vi "Yellow to Red 2.vi"   [LabVIEW 2019]
uses:
  Global Var.vi
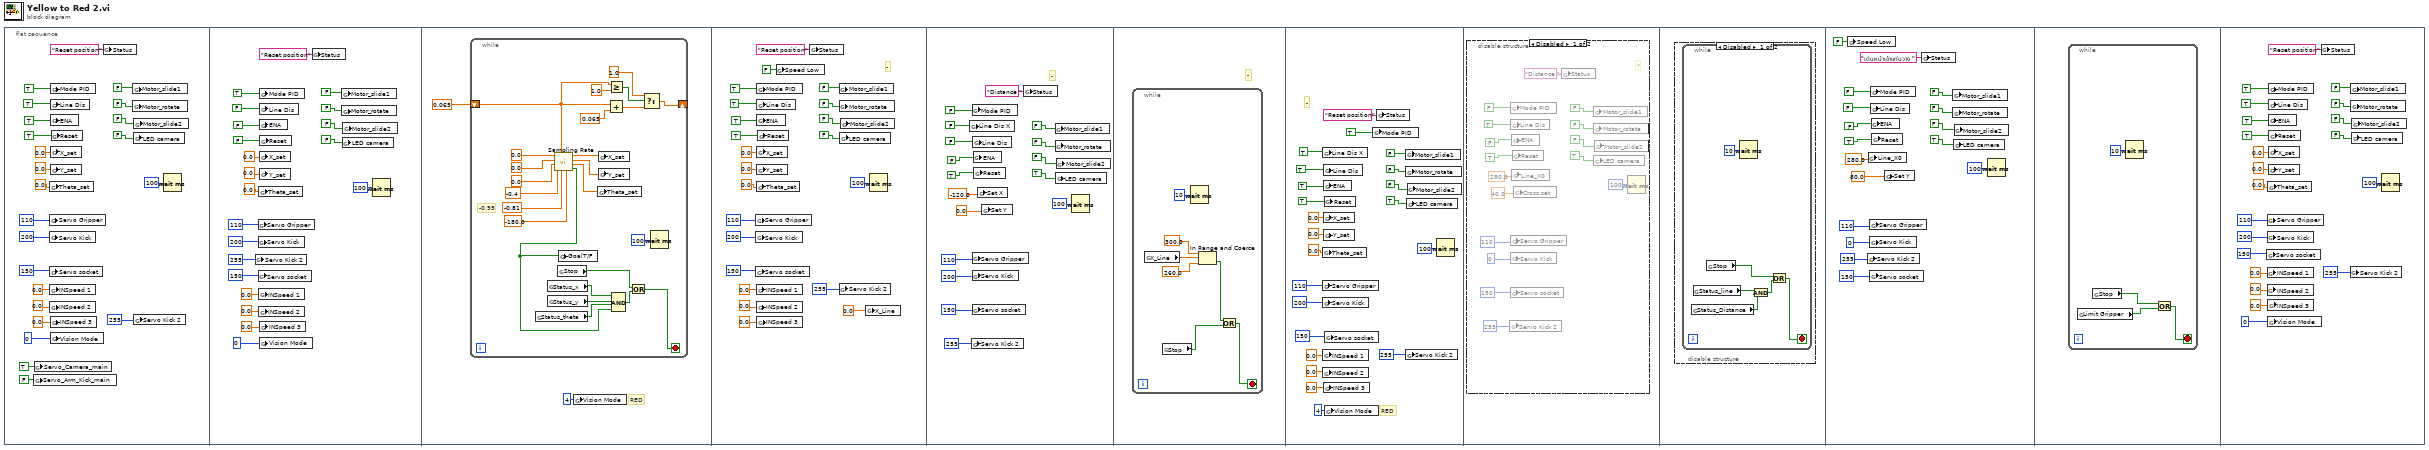
[diagram p0: block diagram]
diagram:
  n1 = flat-sequence {
    frame #0 {
      n2 = global write "Global Var.vi" "Servo_Arm_Kick_main"(FALSE ("Mode PID")) -> ()
      n3 = global write "Global Var.vi" "Servo_Camera_main"(TRUE ("Mode PID")) -> ()
      n4 = global write "Global Var.vi" "Servo Gripper"(u8 110 ("Servo Camera")) -> ()
      n5 = global write "Global Var.vi" "Servo Kick"(u8 200 ("Servo Camera")) -> ()
      n6 = global write "Global Var.vi" "Servo socket"(u8 150 ("Servo Camera")) -> ()
      n7 = global write "Global Var.vi" "Theta_set"(0.0 ("Theta_set")) -> ()
      n8 = global write "Global Var.vi" "INSpeed 1"(0.0 ("X_set")) -> ()
      n9 = global write "Global Var.vi" "INSpeed 2"(0.0 ("Y_set")) -> ()
      n10 = global write "Global Var.vi" "Mode PID"(TRUE ("Mode PID")) -> ()
      n11 = global write "Global Var.vi" "Line Dis"(TRUE ("Mode PID")) -> ()
      n12 = global write "Global Var.vi" "ENA"(TRUE ("ENA")) -> ()
      n13 = global write "Global Var.vi" "X_set"(0.0 ("X_set")) -> ()
      n14 = global write "Global Var.vi" "Y_set"(0.0 ("Y_set")) -> ()
      n15 = global write "Global Var.vi" "INSpeed 3"(0.0 ("Theta_set")) -> ()
      n16 = global write "Global Var.vi" "Vision Mode"(i16 0 ("Vision Mode")) -> ()
      n17 = global write "Global Var.vi" "Reset"(TRUE ("ENA")) -> ()
      n18 = global write "Global Var.vi" "Status"("Reset position" ("Status")) -> ()
      n19 = global write "Global Var.vi" "Motor_slide1"(FALSE ("Mode PID")) -> ()
      n20 = global write "Global Var.vi" "Motor_rotate"(FALSE ("ENA")) -> ()
      n21 = global write "Global Var.vi" "LED camera"(FALSE ("LED camera")) -> ()
      n22 = global write "Global Var.vi" "Motor_slide2"(FALSE ("ENA")) -> ()
      n23 = global write "Global Var.vi" "Servo Kick 2"(u8 255 ("Servo Camera")) -> ()
      n24 = Wait (ms)(milliseconds to wait=u32 100) -> ()  [unwired: 1 out]
    }
    frame #1 {
      n25 = global write "Global Var.vi" "Servo Kick 2"(u8 255 ("Servo Camera")) -> ()
      n26 = global write "Global Var.vi" "Servo Gripper"(u8 110 ("Servo Camera")) -> ()
      n27 = global write "Global Var.vi" "Servo Kick"(u8 200 ("Servo Camera")) -> ()
      n28 = global write "Global Var.vi" "Servo socket"(u8 150 ("Servo Camera")) -> ()
      n29 = global write "Global Var.vi" "Theta_set"(0.0 ("Theta_set")) -> ()
      n30 = global write "Global Var.vi" "INSpeed 1"(0.0 ("X_set")) -> ()
      n31 = global write "Global Var.vi" "INSpeed 2"(0.0 ("Y_set")) -> ()
      n32 = global write "Global Var.vi" "Mode PID"(TRUE ("Mode PID")) -> ()
      n33 = global write "Global Var.vi" "Line Dis"(FALSE ("Mode PID")) -> ()
      n34 = global write "Global Var.vi" "ENA"(FALSE ("ENA")) -> ()
      n35 = global write "Global Var.vi" "X_set"(0.0 ("X_set")) -> ()
      n36 = global write "Global Var.vi" "Y_set"(0.0 ("Y_set")) -> ()
      n37 = global write "Global Var.vi" "INSpeed 3"(0.0 ("Theta_set")) -> ()
      n38 = global write "Global Var.vi" "Vision Mode"(i16 0 ("Vision Mode")) -> ()
      n39 = global write "Global Var.vi" "Reset"(FALSE ("ENA")) -> ()
      n40 = global write "Global Var.vi" "Status"("Reset position" ("Status")) -> ()
      n41 = global write "Global Var.vi" "Motor_slide1"(FALSE ("Mode PID")) -> ()
      n42 = global write "Global Var.vi" "Motor_rotate"(FALSE ("ENA")) -> ()
      n43 = global write "Global Var.vi" "LED camera"(FALSE ("LED camera")) -> ()
      n44 = global write "Global Var.vi" "Motor_slide2"(FALSE ("ENA")) -> ()
      n45 = Wait (ms)(milliseconds to wait=u32 100) -> ()  [unwired: 1 out]
    }
    frame #2 {
      # "RED"
      n46 = while {
        shift-right: [w49] -> _
        shift-left: 0.065 -> [w47]
        stop <- w66 stop-if-true
        # "-0.95"
        n47 = global read "Global Var.vi" "Status_theta"() -> (w68:bool)
        n48 = global read "Global Var.vi" "Status_x"() -> (w69:bool)
        n49 = global read "Global Var.vi" "Status_y"() -> (w70:bool)
        n50 = call "Sampling Rate.vi"("input a1"=-180.0, "input y1"=-0.81, "T(0-1)"=w47, "input x1"=-0.4, "input a0"=0.0, "input y0"=0.0, "input x0"=0.0) -> ("GoalT/F"=w54:bool, "a_output"=w61:dbl, "y_output"=w62:dbl, "x_output"=w63:dbl)  [unwired: 1 in]
        n51 = global read "Global Var.vi" "Stop"() -> (w64:bool)
        n52 = global write "Global Var.vi" "GoalT/F"(w54) -> ()
        n53 = global write "Global Var.vi" "Theta_set"(w61) -> ()
        n54 = global write "Global Var.vi" "X_set"(w63) -> ()
        n55 = global write "Global Var.vi" "Y_set"(w62) -> ()
        n56 = Add(x=w47, y=0.065) -> (x+y=w52:dbl)
        n57 = Greater Or Equal?(x=w47, y=1.0) -> (x >= y?=w51:bool)
        n58 = Compound Arithmetic op=AND(w69, w70, w68, w54) -> (w65:bool)
        n59 = Or(x=w64, y=w65) -> (x .or. y?=w66:bool)
        n60 = Select(t=1.0, s=w51, f=w52) -> (s? t:f=w49:dbl)
        n61 = Wait (ms)(milliseconds to wait=u32 100) -> ()  [unwired: 1 out]
      }
      n62 = global write "Global Var.vi" "Vision Mode"(i16 4 ("Vision Mode")) -> ()
    }
    frame #3 {
      # "-"
      n63 = global write "Global Var.vi" "Servo Gripper"(u8 110 ("Servo Camera")) -> ()
      n64 = global write "Global Var.vi" "Servo Kick"(u8 200 ("Servo Camera")) -> ()
      n65 = global write "Global Var.vi" "Servo socket"(u8 150 ("Servo Camera")) -> ()
      n66 = global write "Global Var.vi" "Theta_set"(0.0 ("Theta_set")) -> ()
      n67 = global write "Global Var.vi" "INSpeed 1"(0.0 ("X_set")) -> ()
      n68 = global write "Global Var.vi" "INSpeed 2"(0.0 ("Y_set")) -> ()
      n69 = global write "Global Var.vi" "Mode PID"(TRUE ("Mode PID")) -> ()
      n70 = global write "Global Var.vi" "Line Dis"(TRUE ("Mode PID")) -> ()
      n71 = global write "Global Var.vi" "ENA"(TRUE ("ENA")) -> ()
      n72 = global write "Global Var.vi" "X_set"(0.0 ("X_set")) -> ()
      n73 = global write "Global Var.vi" "Y_set"(0.0 ("Y_set")) -> ()
      n74 = global write "Global Var.vi" "INSpeed 3"(0.0 ("Theta_set")) -> ()
      n75 = global write "Global Var.vi" "Reset"(TRUE ("ENA")) -> ()
      n76 = global write "Global Var.vi" "Speed Low"(FALSE ("Speed Low")) -> ()
      n77 = global write "Global Var.vi" "Status"("Reset position" ("Status")) -> ()
      n78 = global write "Global Var.vi" "Motor_slide1"(FALSE ("Mode PID")) -> ()
      n79 = global write "Global Var.vi" "Motor_rotate"(FALSE ("ENA")) -> ()
      n80 = global write "Global Var.vi" "Servo Kick 2"(u8 255 ("Servo Camera")) -> ()
      n81 = global write "Global Var.vi" "LED camera"(FALSE ("LED camera")) -> ()
      n82 = global write "Global Var.vi" "Motor_slide2"(FALSE ("ENA")) -> ()
      n83 = global write "Global Var.vi" "X_Line"(0.0 ("X_set")) -> ()
      n84 = Wait (ms)(milliseconds to wait=u32 100) -> ()  [unwired: 1 out]
    }
    frame #4 {
      # "-"
      n85 = global write "Global Var.vi" "Line Dis X"(FALSE ("Mode PID")) -> ()
      n86 = global write "Global Var.vi" "Servo Kick 2"(u8 255 ("Servo Camera")) -> ()
      n87 = global write "Global Var.vi" "Mode PID"(FALSE ("Mode PID")) -> ()
      n88 = global write "Global Var.vi" "Servo Gripper"(u8 110 ("Servo Camera")) -> ()
      n89 = global write "Global Var.vi" "Servo Kick"(u8 200 ("Servo Camera")) -> ()
      n90 = global write "Global Var.vi" "Servo socket"(u8 150 ("Servo Camera")) -> ()
      n91 = global write "Global Var.vi" "Line Dis"(FALSE ("Mode PID")) -> ()
      n92 = global write "Global Var.vi" "ENA"(FALSE ("ENA")) -> ()
      n93 = global write "Global Var.vi" "Reset"(TRUE ("ENA")) -> ()
      n94 = global write "Global Var.vi" "Set X"(-120.0 ("Y_set")) -> ()
      n95 = global write "Global Var.vi" "Set Y"(0.0 ("Y_set")) -> ()
      n96 = global write "Global Var.vi" "Status"("Distance " ("Status")) -> ()
      n97 = global write "Global Var.vi" "Motor_slide1"(FALSE ("Mode PID")) -> ()
      n98 = global write "Global Var.vi" "Motor_rotate"(FALSE ("ENA")) -> ()
      n99 = global write "Global Var.vi" "LED camera"(TRUE ("LED camera")) -> ()
      n100 = global write "Global Var.vi" "Motor_slide2"(FALSE ("ENA")) -> ()
      n101 = Wait (ms)(milliseconds to wait=u32 100) -> ()  [unwired: 1 out]
    }
    frame #5 {
      # "-"
      n102 = while {
        stop <- w115 stop-if-true
        n103 = global read "Global Var.vi" "X_Line"() -> (w113:dbl)
        n104 = global read "Global Var.vi" "Stop"() -> (w114:bool)
        n105 = Wait (ms)(milliseconds to wait=u32 10) -> ()  [unwired: 1 out]
        n106 = In Range and Coerce(upper limit=300.0, x=w113, lower limit=260.0) -> (In Range?=w110:bool)  [unwired: 1 out]
        n107 = Or(x=w110, y=w114) -> (x .or. y?=w115:bool)
      }
    }
    frame #6 {
      # "RED"
      # "-"
      n108 = global write "Global Var.vi" "Servo Gripper"(u8 110 ("Servo Camera")) -> ()
      n109 = global write "Global Var.vi" "Servo Kick"(u8 200 ("Servo Camera")) -> ()
      n110 = global write "Global Var.vi" "Line Dis X"(TRUE ("Mode PID")) -> ()
      n111 = global write "Global Var.vi" "Theta_set"(0.0 ("Theta_set")) -> ()
      n112 = global write "Global Var.vi" "INSpeed 1"(0.0 ("X_set")) -> ()
      n113 = global write "Global Var.vi" "INSpeed 2"(0.0 ("Y_set")) -> ()
      n114 = global write "Global Var.vi" "Line Dis"(TRUE ("Mode PID")) -> ()
      n115 = global write "Global Var.vi" "ENA"(TRUE ("ENA")) -> ()
      n116 = global write "Global Var.vi" "X_set"(0.0 ("X_set")) -> ()
      n117 = global write "Global Var.vi" "Y_set"(0.0 ("Y_set")) -> ()
      n118 = global write "Global Var.vi" "INSpeed 3"(0.0 ("Theta_set")) -> ()
      n119 = global write "Global Var.vi" "Reset"(TRUE ("ENA")) -> ()
      n120 = global write "Global Var.vi" "Servo socket"(u8 150 ("Servo Camera")) -> ()
      n121 = global write "Global Var.vi" "Vision Mode"(i16 4 ("Vision Mode")) -> ()
      n122 = global write "Global Var.vi" "Mode PID"(TRUE ("Mode PID")) -> ()
      n123 = global write "Global Var.vi" "Status"("Reset position" ("Status")) -> ()
      n124 = global write "Global Var.vi" "Motor_slide1"(FALSE ("Mode PID")) -> ()
      n125 = global write "Global Var.vi" "Motor_rotate"(FALSE ("ENA")) -> ()
      n126 = global write "Global Var.vi" "Servo Kick 2"(u8 255 ("Servo Camera")) -> ()
      n127 = global write "Global Var.vi" "LED camera"(TRUE ("LED camera")) -> ()
      n128 = global write "Global Var.vi" "Motor_slide2"(FALSE ("ENA")) -> ()
      n129 = Wait (ms)(milliseconds to wait=u32 100) -> ()  [unwired: 1 out]
    }
    frame #7 {
      n130 = disable-structure shown="Disabled" {
        frame Disabled {
          # "*"
          n131 = global write "Global Var.vi" "Servo Kick 2"(u8 255 ("Servo Camera")) -> ()
          n132 = global write "Global Var.vi" "Servo Gripper"(u8 110 ("Servo Camera")) -> ()
          n133 = global write "Global Var.vi" "Servo Kick"(u8 0 ("Servo Camera")) -> ()
          n134 = global write "Global Var.vi" "Servo socket"(u8 150 ("Servo Camera")) -> ()
          n135 = global write "Global Var.vi" "Mode PID"(FALSE ("Mode PID")) -> ()
          n136 = global write "Global Var.vi" "Line Dis"(TRUE ("Mode PID")) -> ()
          n137 = global write "Global Var.vi" "ENA"(FALSE ("ENA")) -> ()
          n138 = global write "Global Var.vi" "Line_X0"(280.0 ("Y_set")) -> ()
          n139 = global write "Global Var.vi" "Reset"(TRUE ("ENA")) -> ()
          n140 = global write "Global Var.vi" "Cross set"(40.0 ("Y_set")) -> ()
          n141 = global write "Global Var.vi" "Status"("Distance " ("Status")) -> ()
          n142 = global write "Global Var.vi" "Motor_slide1"(FALSE ("Mode PID")) -> ()
          n143 = global write "Global Var.vi" "Motor_rotate"(FALSE ("ENA")) -> ()
          n144 = global write "Global Var.vi" "LED camera"(TRUE ("LED camera")) -> ()
          n145 = global write "Global Var.vi" "Motor_slide2"(FALSE ("ENA")) -> ()
          n146 = Wait (ms)(milliseconds to wait=u32 100) -> ()  [unwired: 1 out]
        }
        frame Enabled {
        }
      }
    }
    frame #8 {
      n147 = disable-structure shown="Disabled" {
        frame Disabled {
          n148 = while {
            stop <- w159 stop-if-true
            n149 = global read "Global Var.vi" "Status_Distance"() -> (w155:bool)
            n150 = global read "Global Var.vi" "Status_line"() -> (w156:bool)
            n151 = global read "Global Var.vi" "Stop"() -> (w158:bool)
            n152 = Wait (ms)(milliseconds to wait=u32 10) -> ()  [unwired: 1 out]
            n153 = And(x=w156, y=w155) -> (x .and. y?=w157:bool)
            n154 = Or(x=w158, y=w157) -> (x .or. y?=w159:bool)
          }
        }
        frame Enabled {
        }
      }
    }
    frame #9 {
      n155 = global write "Global Var.vi" "Speed Low"(FALSE ("Speed Low")) -> ()
      n156 = global write "Global Var.vi" "Servo Kick 2"(u8 255 ("Servo Camera")) -> ()
      n157 = global write "Global Var.vi" "Line_X0"(280.0 ("Y_set")) -> ()
      n158 = global write "Global Var.vi" "Servo Gripper"(u8 110 ("Servo Camera")) -> ()
      n159 = global write "Global Var.vi" "Servo Kick"(u8 0 ("Servo Camera")) -> ()
      n160 = global write "Global Var.vi" "Servo socket"(u8 150 ("Servo Camera")) -> ()
      n161 = global write "Global Var.vi" "Mode PID"(FALSE ("Mode PID")) -> ()
      n162 = global write "Global Var.vi" "Line Dis"(FALSE ("Mode PID")) -> ()
      n163 = global write "Global Var.vi" "ENA"(FALSE ("ENA")) -> ()
      n164 = global write "Global Var.vi" "Reset"(TRUE ("ENA")) -> ()
      n165 = global write "Global Var.vi" "Set Y"(80.0 ("Y_set")) -> ()
      n166 = global write "Global Var.vi" "Status"("เดินหน้าเข้าแท่นวาง " ("Status")) -> ()
      n167 = global write "Global Var.vi" "Motor_slide1"(FALSE ("Mode PID")) -> ()
      n168 = global write "Global Var.vi" "Motor_rotate"(FALSE ("ENA")) -> ()
      n169 = global write "Global Var.vi" "LED camera"(TRUE ("LED camera")) -> ()
      n170 = global write "Global Var.vi" "Motor_slide2"(FALSE ("ENA")) -> ()
      n171 = Wait (ms)(milliseconds to wait=u32 100) -> ()  [unwired: 1 out]
    }
    frame #10 {
      n172 = while {
        stop <- w180 stop-if-true
        n173 = global read "Global Var.vi" "Limit Gripper"() -> (w178:bool)
        n174 = global read "Global Var.vi" "Stop"() -> (w179:bool)
        n175 = Wait (ms)(milliseconds to wait=u32 10) -> ()  [unwired: 1 out]
        n176 = Or(x=w179, y=w178) -> (x .or. y?=w180:bool)
      }
    }
    frame #11 {
      n177 = global write "Global Var.vi" "Servo socket"(u8 150 ("Servo Camera")) -> ()
      n178 = global write "Global Var.vi" "Servo Gripper"(u8 110 ("Servo Camera")) -> ()
      n179 = global write "Global Var.vi" "Servo Kick"(u8 200 ("Servo Camera")) -> ()
      n180 = global write "Global Var.vi" "INSpeed 1"(0.0 ("X_set")) -> ()
      n181 = global write "Global Var.vi" "INSpeed 2"(0.0 ("Y_set")) -> ()
      n182 = global write "Global Var.vi" "Theta_set"(0.0 ("Theta_set")) -> ()
      n183 = global write "Global Var.vi" "INSpeed 3"(0.0 ("Theta_set")) -> ()
      n184 = global write "Global Var.vi" "Vision Mode"(i16 0 ("Vision Mode")) -> ()
      n185 = global write "Global Var.vi" "Mode PID"(TRUE ("Mode PID")) -> ()
      n186 = global write "Global Var.vi" "Line Dis"(TRUE ("Mode PID")) -> ()
      n187 = global write "Global Var.vi" "ENA"(TRUE ("ENA")) -> ()
      n188 = global write "Global Var.vi" "X_set"(0.0 ("X_set")) -> ()
      n189 = global write "Global Var.vi" "Y_set"(0.0 ("Y_set")) -> ()
      n190 = global write "Global Var.vi" "Reset"(TRUE ("ENA")) -> ()
      n191 = global write "Global Var.vi" "Status"("Reset position" ("Status")) -> ()
      n192 = global write "Global Var.vi" "Servo Kick 2"(u8 255 ("Servo Camera")) -> ()
      n193 = global write "Global Var.vi" "Motor_slide1"(FALSE ("Mode PID")) -> ()
      n194 = global write "Global Var.vi" "Motor_rotate"(FALSE ("ENA")) -> ()
      n195 = global write "Global Var.vi" "LED camera"(FALSE ("LED camera")) -> ()
      n196 = global write "Global Var.vi" "Motor_slide2"(FALSE ("ENA")) -> ()
      n197 = Wait (ms)(milliseconds to wait=u32 100) -> ()  [unwired: 1 out]
    }
  }
